vi "LeerBD_interno.vi"(8 "error in (no error)":errorcluster) -> (0 "error out":errorcluster, 2 "BD":T1={"frec_referencia"=98.0, "niv_presion_son_ref"=97.0, "Incertidumbre"=["1", "1", "1", "1", "1", "1", "1", "1", "1", "1"], "Tol +"=["2,0", "1,5", "1,5", "1,4", "1,4", "1,1", "1,6", "1,6", "2,1", "3,5"], "Tol -"=["-2,0", "-1,5", "-1,5", "-1,4", "-1,4", "-1,1", "-1,6", "-1,6", "-2,1", "-3,5"], "Referencia(dB)"=["95", "94", "94", "94", "96", "95", "94", "96", "95", "94"], "Frecuencias(Hz)"=["95", "94", "94", "94", "96", "95", "94", "96", "95", "94"], "vol_enviado_CAM"=0.0, "CorreccionMic"=["95", "94", "94", "94", "96", "95", "94", "96", "95", "94"]}, 3 "Prueba02 out":refnum<class "Prueba02.lvclass">)   [LabVIEW 2019, in "Prueba031.lvclass"]
uses:
  Prueba031.lvclass
  Prueba02/Prueba02.lvclass
  Controles/BD.ctl
  Base de Datos/SQLiteConnector/SQLiteConnection.lvclass
  Base de Datos/Base de Datos.lvclass
panel:
  in  "Tipo Equipo":enum16{"Sonometro", "Calibrador", "Dosimetro"}(ring)
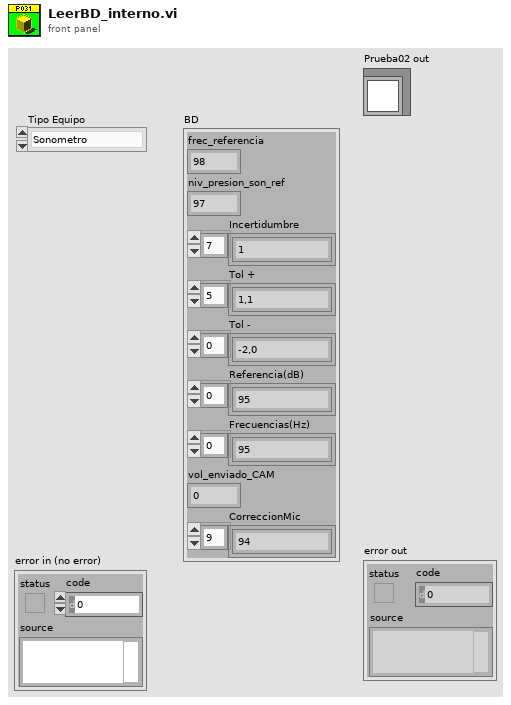
[diagram p1: front panel]
types:
  T1 = typedef "Prueba031.lvclass/BD.ctl" = cluster{"frec_referencia":dbl, "niv_presion_son_ref":dbl, "Incertidumbre":string[], "Tol +":string[], "Tol -":string[], "Referencia(dB)":string[], "Frecuencias(Hz)":string[], "vol_enviado_CAM":dbl, "CorreccionMic":string[]}
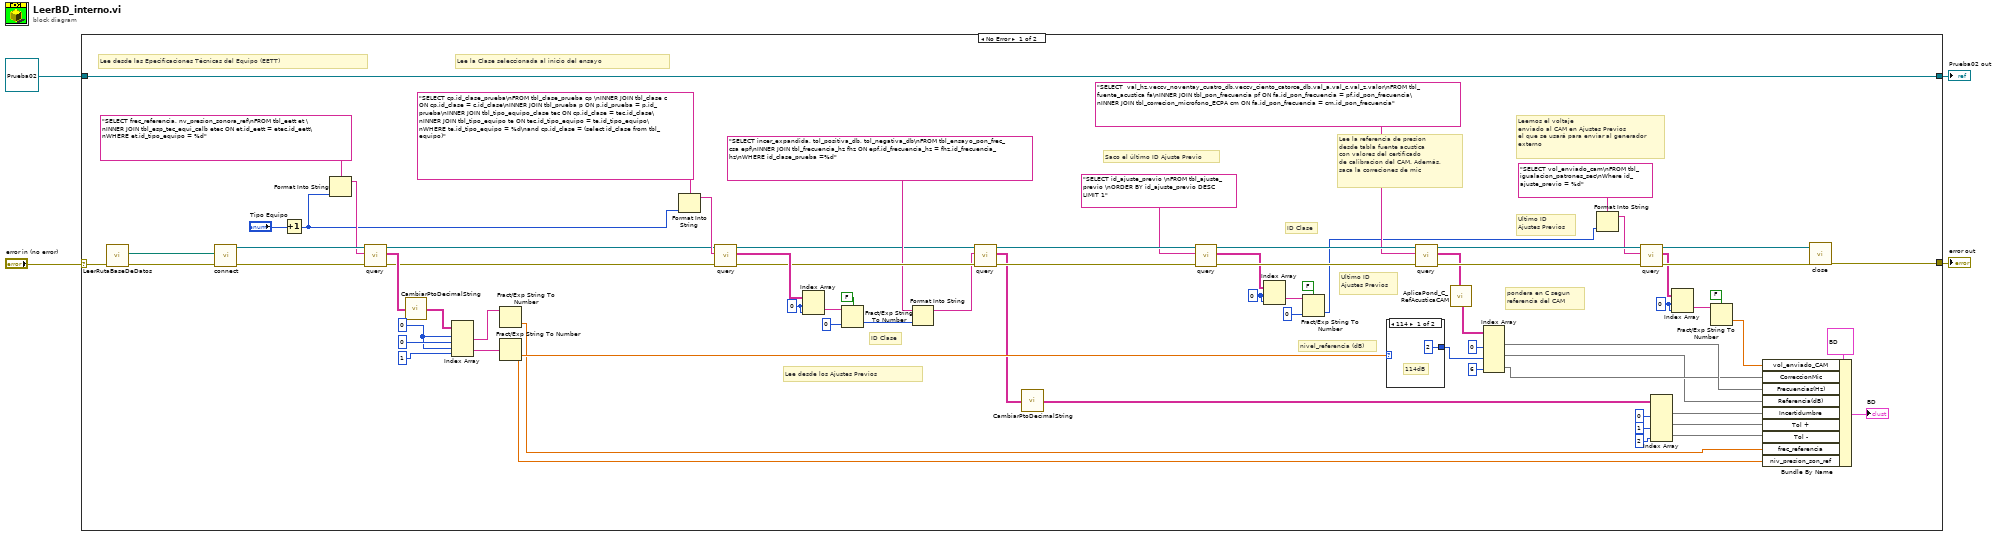
[diagram p0: block diagram]
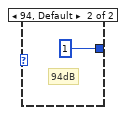
[diagram p2: hidden frame]
diagram:
  n1 = case shown="No Error" "error in (no error)" {
    selector: "error in (no error)" -> [w71 w83]
    tunnel: [w55 w83] -> w3
    tunnel: [w79 w82] -> w1
    tunnel: refnum<class "Prueba02.lvclass"> refnum ("Prueba02 in") -> [w79 w82]
    frame No Error {
      w16 = 0 ("index (row)")
      w29 = 0 ("index (row)")
      w61 = 0 ("index (row)")
      w54 = 0 ("index (row)")
      # "pondera en C segun \nreferencia del CAM"
      # "Ultimo ID\nAjustes Previos"
      # "Ultimo ID\nAjustes Previos"
      # "ID Clase"
      # "Leemos el voltaje\nenviado al CAM en Ajustes Previos\nel que se usará para enviar al generador\nexterno"
      # "Lee la referencia de presion\ndesde tabla fuente acustica\ncon valores del certificado\nde calibracion del CAM. Además,\nsaca la correciones de mic"
      # "ID Clase"
      # "Saco el último ID Ajuste Previo"
      # "nivel_referencia (dB)"
      # "Lee desde los Ajustes Previos"
      # "Lee la Clase seleccionada al inicio del ensayo"
      # "Lee desde las Epecificaciones Técnicas del Equipo (EETT)"
      n2 = call "LeerRutaBaseDeDatos.vi"("error in (no error)"=w71) -> ("error out"=w74:errorcluster, "Database Path"=w73:path)  [unwired: 9 in]
      n3 = call "connect.vi"("error in (no error)"=w74, "Database Path"=w73) -> ("error out"=w76:errorcluster, "object out"=w77:refnum<class "SQLiteConnection.lvclass">)  [unwired: 8 in]
      n4 = Increment(x="Tipo Equipo") -> (x+1=w48:enum16{"Sonometro", "Calibrador", "Dosimetro"})
      n5 = Format Into String(format string="SELECT frec_referencia, nv_presion_sonora_ref\nFROM tbl_eett et \nINNER JOIN tbl_esp_tec_equi_calb etec ON et.id_eett = etec.id_eett\nWHERE et.id_tipo_equipo = %d", w48) -> (resulting string=w75:string)  [unwired: 2 in, 1 out]
      n6 = call "query.vi"("error in (no error)"=w76, "SQL Statement"=w75, "object in"=w77) -> ("error out"=w62:errorcluster, "result"=w66:string[][], "object out"=w63:refnum<class "SQLiteConnection.lvclass">)  [unwired: 5 in, 1 out]
      n7 = call "CambiarPtoDecimalString.vi"("result"=w66) -> ("result out"=w5:string[][])
      n8 = Index Array(array=w5, index (row) #1=w54, index (col) #1=0 ("disabled index (col)"), index (row) #2=w54, index (col) #2=1 ("disabled index (col)")) -> (element #1=w68:string, element #2=w67:string)
      n9 = Fract/Exp String To Number(string=w68) -> (number=w37:dbl)  [unwired: 3 in, 1 out]
      n10 = Fract/Exp String To Number(string=w67) -> (number=w47:dbl)  [unwired: 3 in, 1 out]
      n11 = Format Into String(format string="SELECT cp.id_clase_prueba\nFROM tbl_clase_prueba cp \nINNER JOIN tbl_clase c ON cp.id_clase = c.id_clase\nINNER JOIN tbl_prueba p ON p.id_prueba = p.id_prueba\nINNER JOIN tbl_tipo_equipo_clase tec ON cp.id_clase = tec.id_clase\nINNER JOIN tbl_tipo_equipo te ON tec.id_tipo_equipo = te.id_tipo_equipo\nWHERE te.id_tipo_equipo = %d\nand cp.id_clase = (select id_clase from tbl_equipo)", w48) -> (resulting string=w64:string)  [unwired: 2 in, 1 out]
      n12 = call "query.vi"("error in (no error)"=w62, "SQL Statement"=w64, "object in"=w63) -> ("error out"=w56:errorcluster, "result"=w57:string[][], "object out"=w51:refnum<class "SQLiteConnection.lvclass">)  [unwired: 5 in, 1 out]
      n13 = Index Array(array=w57, index (row)=w61, index (col)=w61) -> (element=w59:string)
      n14 = Fract/Exp String To Number(use system decimal point (T)=FALSE, string=w59, default (0 dbl)=0 ("index (row)")) -> (number=w13:i32)  [unwired: 1 in, 1 out]
      n15 = Format Into String(format string="SELECT incer_expandida, tol_positiva_db, tol_negativa_db\nFROM tbl_ensayo_pon_frec_csa epf\nINNER JOIN tbl_frecuencia_hz fhz ON epf.id_frecuencia_hz = fhz.id_frecuencia_hz\nWHERE id_clase_prueba =%d", w13) -> (resulting string=w50:string)  [unwired: 2 in, 1 out]
      n16 = call "query.vi"("error in (no error)"=w56, "SQL Statement"=w50, "object in"=w51) -> ("error out"=w52:errorcluster, "result"=w42:string[][], "object out"=w35:refnum<class "SQLiteConnection.lvclass">)  [unwired: 5 in, 1 out]
      n17 = call "CambiarPtoDecimalString.vi"("result"=w42) -> ("result out"=w6:string[][])
      n18 = call "query.vi"("error in (no error)"=w52, "SQL Statement"="SELECT id_ajuste_previo \nFROM tbl_ajuste_previo \nORDER BY id_ajuste_previo DESC LIMIT 1" ("format string"), "object in"=w35) -> ("error out"=w36:errorcluster, "result"=w28:string[][], "object out"=w34:refnum<class "SQLiteConnection.lvclass">)  [unwired: 5 in, 1 out]
      n19 = Index Array(array=w28, index (row)=w29, index (col)=w29) -> (element=w31:string)
      n20 = Fract/Exp String To Number(use system decimal point (T)=FALSE, string=w31, default (0 dbl)=0 ("index (row)")) -> (number=w19:i32)  [unwired: 1 in, 1 out]
      n21 = case shown="114" w47 {
        tunnel: [2 ("disabled index (col)") 1 ("disabled index (col)")] -> w14
        frame 114 {
          # "114dB"
        }
        frame 94, Default {
          # "94dB"
        }
      }
      n22 = call "query.vi"("error in (no error)"=w36, "SQL Statement"="SELECT  val_hz,veccv_noventay_cuatro_db,veccv_ciento_catorce_db,val_a,val_c,val_z,valor\nFROM tbl_fuente_acustica fa\nINNER JOIN tbl_pon_frecuencia pf ON fa.id_pon_frecuencia = pf.id_pon_frecuencia\nINNER JOIN tbl_correcion_microfono_ECPA cm ON fa.id_pon_frecuencia = cm.id_pon_frecuencia" ("format string"), "object in"=w34) -> ("error out"=w49:errorcluster, "result"=w9:string[][], "object out"=w23:refnum<class "SQLiteConnection.lvclass">)  [unwired: 5 in, 1 out]
      n23 = call "AplicaPond_C_RefAcusticaCAM.vi"("result"=w9) -> ("output array"=w8:string[][])
      n24 = Index Array(array=w8, index (col) #1=0 ("disabled index (col)"), index (col) #2=w14, index (col) #3=6 ("index (col)")) -> (element #1=w25:string[], element #2=w7:string[], element #3=w10:string[])  [unwired: 3 in]
      n25 = Format Into String(format string="SELECT vol_enviado_cam\nFROM tbl_igualacion_patrones_sec\nWhere id_ajuste_previo = %d", w19) -> (resulting string=w20:string)  [unwired: 2 in, 1 out]
      n26 = call "query.vi"("error in (no error)"=w49, "SQL Statement"=w20, "object in"=w23) -> ("error out"=w24:errorcluster, "result"=w15:string[][], "object out"=w22:refnum<class "SQLiteConnection.lvclass">)  [unwired: 5 in, 1 out]
      n27 = Index Array(array=w6, index (col) #1=0 ("disabled index (col)"), index (col) #2=1 ("index (col)"), index (col) #3=2 ("index (col)")) -> (element #1=w45:string[], element #2=w44:string[], element #3=w43:string[])  [unwired: 3 in]
      n28 = Index Array(array=w15, index (row)=w16, index (col)=w16) -> (element=w18:string)
      n29 = Fract/Exp String To Number(use system decimal point (T)=FALSE, string=w18) -> (number=w12:dbl)  [unwired: 2 in, 1 out]
      n30 = Bundle By Name(cluster=T1 {"frec_referencia"=98.0, "niv_presion_son_ref"=97.0, "Incertidumbre"=["1", "1", "1", "1", "1", "1", "1", "1", "1", "1"], "Tol +"=["2,0", "1,5", "1,5", "1,4", "1,4", "1,1", "1,6", "1,6", "2,1", "3,5"], "Tol -"=["-2,0", "-1,5", "-1,5", "-1,4", "-1,4", "-1,1", "-1,6", "-1,6", "-2,1", "-3,5"], "Referencia(dB)"=["95", "94", "94", "94", "96", "95", "94", "96", "95", "94"], "Frecuencias(Hz)"=["95", "94", "94", "94", "96", "95", "94", "96", "95", "94"], "vol_enviado_CAM"=0.0, "CorreccionMic"=["95", "94", "94", "94", "96", "95", "94", "96", "95", "94"]} ("BD"), "vol_enviado_CAM"=w12, "CorreccionMic"=w10, "Frecuencias(Hz)"=w25, "Referencia(dB)"=w7, "Incertidumbre"=w45, "Tol +"=w44, "Tol -"=w43, "frec_referencia"=w37, "niv_presion_son_ref"=w47) -> (→"BD":T1)
      n31 = call-dynamic "close.vi"("error in (no error)"=w24, "object in"=w22) -> ("error out"=w55:errorcluster)  [unwired: 8 in, 1 out]
    }
    frame Error {
    }
  }
  "error out" <- w3
  "Prueba02 out" <- w1
